vi "Write_txt.vi"(8 "error in":errorcluster, 9 "text":string, 10 "filename.txt":string="error_log.txt", 11 "base path":path) -> (0 "error out":errorcluster)   [LabVIEW 2017]
doc: "This SubVI open or create txt file in certain directory"
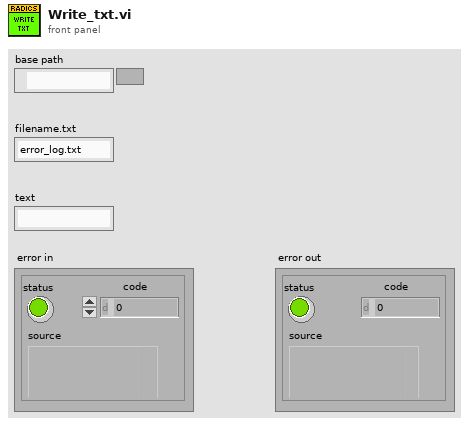
[diagram p1: front panel]
types:
  T1 = enum16{"open", "replace", "create", "open or create", "replace or create", "replace or create with confirmation"}
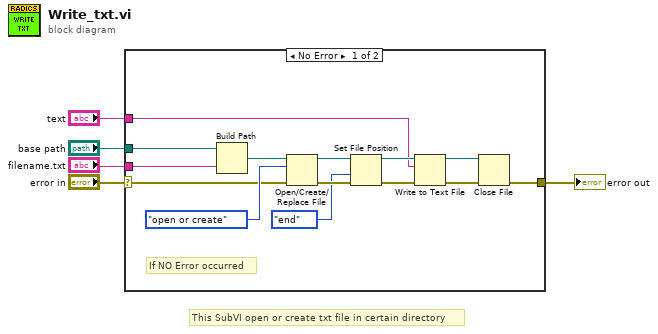
[diagram p0: block diagram]
diagram:
  # "This SubVI open or create txt file in certain directory"
  n1 = case shown="No Error" "error in" {
    selector: "error in" -> [w10 w20]
    tunnel: [w9 w20] -> w4
    tunnel: "filename.txt" -> [w8 _]
    tunnel: "base path" -> [w7 _]
    tunnel: "text" -> [w6 _]
    frame No Error {
      # "If NO Error occurred"
      n2 = Build Path(base path=w7, name or relative path=w8) -> (appended path=w19:path)
      n3 = Open/Create/Replace File(file path (use dialog)=w19, error in=w10, operation (0:open)=T1."open or create") -> (refnum out=w17:refnum<file>, error out=w16:errorcluster)  [unwired: 3 in, 1 out]
      n4 = Set File Position(refnum=w17, from (0:start)=enum16{"start", "end", "current"}."end", error in=w16) -> (refnum out=w15:refnum<file>, error out=w14:errorcluster)  [unwired: 1 in]
      n5 = Write to Text File(file (use dialog)=w15, text=w6, error in=w14) -> (refnum out=w12:refnum<file>, error out=w13:errorcluster)  [unwired: 1 in, 1 out]
      n6 = Close File(refnum=w12, error in=w13) -> (error out=w9:errorcluster)  [unwired: 1 out]
    }
    frame Error {
      # "If any error occurred"
    }
  }
  "error out" <- w4
